vi "Manager.vi"(7 "Action":T1, 8 "Error In":errorcluster, 11 "Value In":variant) -> (0 "Error Out":errorcluster)   [LabVIEW 2017, in "Logger.lvlib"]
uses:
  Logger.lvlib
  Action.ctl
  Public/Controls/Statement.ctl
  Public/Controls/Tag.ctl
  Find.vi
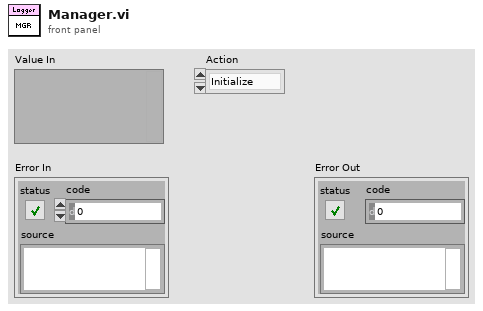
[diagram p1: front panel]
types:
  T1 = typedef "Logger.lvlib/Action.ctl" = enum16{"Initialize", "Register", "Log", "Unregister", "Set Level", "Shutdown"}
  T2 = typedef "Logger.lvlib/Statement.ctl" = cluster{"Time Stamp":timestamp, "Tag":T3, "Source":string, "Message":string}
  T3 = typedef "Logger.lvlib/Tag.ctl" = enum16{"Fatal", "Error", "Warn", "Info", "Debug", "Trace"}
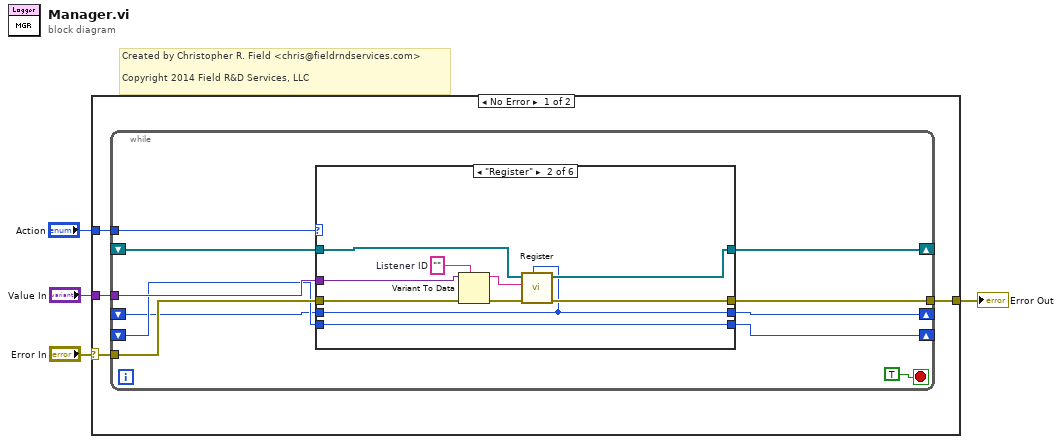
[diagram p0: block diagram]
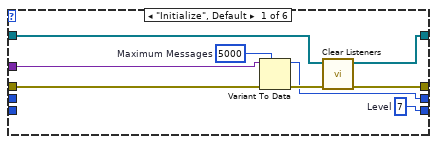
[diagram p2: hidden frame]
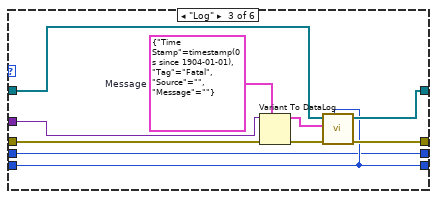
[diagram p3: hidden frame]
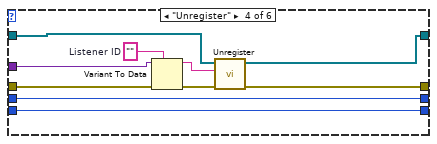
[diagram p4: hidden frame]
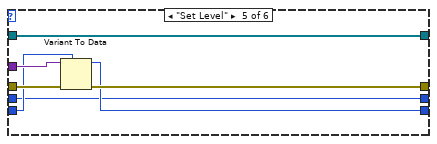
[diagram p5: hidden frame]
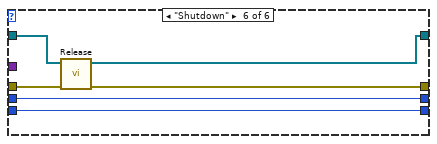
[diagram p6: hidden frame]
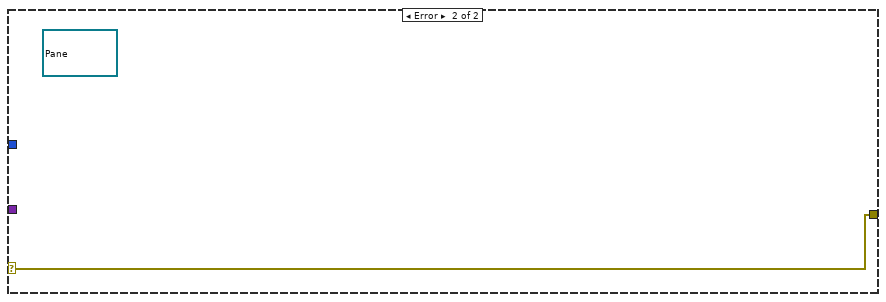
[diagram p7: hidden frame]
diagram:
  # "Created by Christopher R. Field <chris@fieldrndservices.com>\n\nCopyright 2014 Field R&D Services, LLC"
  n1 = case shown="No Error" "Error In" {
    selector: "Error In" -> [w7 w72]
    tunnel: [w6 w72] -> w3
    tunnel: "Action" -> [w8 _]
    tunnel: "Value In" -> [w5 _]
    frame No Error {
      n2 = while {
        tunnel: w8 -> [w18]
        tunnel: w7 -> [w17]
        tunnel: [w16] -> w6
        shift-right: [w15] -> _
        shift-left: _ -> [w14]
        tunnel: w5 -> [w13]
        shift-right: [w12] -> _
        shift-left: _ -> [w11]
        shift-right: [w10] -> _
        shift-left: _ -> [w9]
        stop <- TRUE stop-if-true
        n3 = case shown="\"Register\"" w18 {
          tunnel: w17 -> [w26 w35 w47 w57 w64 w70]
          tunnel: [w25 w38 w48 w51 w62 w69] -> w16
          tunnel: [w28 w37 w42 w52 w63 w68] -> w15
          tunnel: w14 -> [w27 w32 w43 w53 w63 w71]
          tunnel: w13 -> [w22 w36 w45 w58 w65 _]
          tunnel: [w24 w30 w40 w50 w60 w67] -> w12
          tunnel: w11 -> [_ w30 w40 w50 w61 w67]
          tunnel: [w20 w29 w39 w49 w59 w66] -> w10
          tunnel: w9 -> [_ w29 w39 w49 w59 w66]
          frame "Initialize", Default {
            w21 = 5000  # Maximum Messages
            w24 = u8 7  # Level
            n4 = Variant To Data(error in=w26, type=w21, Variant=w22) -> (data=w20:i32, error out=w23:errorcluster)
            n5 = call "Clear Listeners.vi"("Error In"=w23, "Listeners In"=w27) -> ("Error Out"=w25:errorcluster, "Listeners Out"=w28:refnum<queue>[])  [unwired: 8 in]
          }
          frame "Register" {
            w33 = ""  # Listener ID
            n6 = Variant To Data(error in=w35, type=w33, Variant=w36) -> (data=w31:string, error out=w34:errorcluster)
            n7 = call "Register.vi"("Maximum Messages"=w29, "Error In"=w34, "Listener ID"=w31, "Listeners In"=w32) -> ("Error Out"=w38:errorcluster, "Listeners Out"=w37:refnum<queue>[])  [unwired: 6 in]
          }
          frame "Log" {
            w44 = T2 {"Time Stamp"=timestamp(0 s since 1904-01-01), "Tag"=enum."Fatal", "Source"="", "Message"=""}  # Message
            n8 = Variant To Data(error in=w47, type=w44, Variant=w45) -> (data=w41:T2, error out=w46:errorcluster)
            n9 = call "Log.vi"("Level"=w40, "Error In"=w46, "Message"=w41, "Listeners In"=w43) -> ("Error Out"=w48:errorcluster, "Listeners Out"=w42:refnum<queue>[])  [unwired: 6 in]
          }
          frame "Unregister" {
            w56 = ""  # Listener ID
            n10 = Variant To Data(error in=w57, type=w56, Variant=w58) -> (data=w54:string, error out=w55:errorcluster)
            n11 = call "Unregister.vi"("Error In"=w55, "Listener ID"=w54, "Listeners In"=w53) -> ("Error Out"=w51:errorcluster, "Listeners Out"=w52:refnum<queue>[])  [unwired: 7 in]
          }
          frame "Set Level" {
            n12 = Variant To Data(error in=w64, type=w61, Variant=w65) -> (data=w60:u8, error out=w62:errorcluster)
          }
          frame "Shutdown" {
            n13 = call "Release.vi"("Error In"=w70, "Listeners In"=w71) -> ("Error Out"=w69:errorcluster, "Listeners Out"=w68:refnum<queue>[])  [unwired: 8 in]
          }
        }
      }
    }
    frame Error {
      (unwired) refnum<user-event> refnum ("Log")
    }
  }
  "Error Out" <- w3
